vi "Analog IO Message - Continuous Pin Report.vi"(8 "error in (no error)":errorcluster, 9 "Enable Continuous Reporting?":bool, 10 "Pin Index":u8 format="%x", 11 "Refnum In":refnum<vi>) -> (0 "error out":errorcluster, 1 "Pin Value":u16, 2 "Pin Index Out":u8, 3 "Refnum Out":refnum<vi>)   [LabVIEW 2020, in "FirmataClient.lvlib"]
doc: "Allows requesting the state of a analog pin."
uses:
  FirmataClient.lvlib
  Controls/FirmataPinModes.ctl
panel:
  out "Pin Voltage":dbl
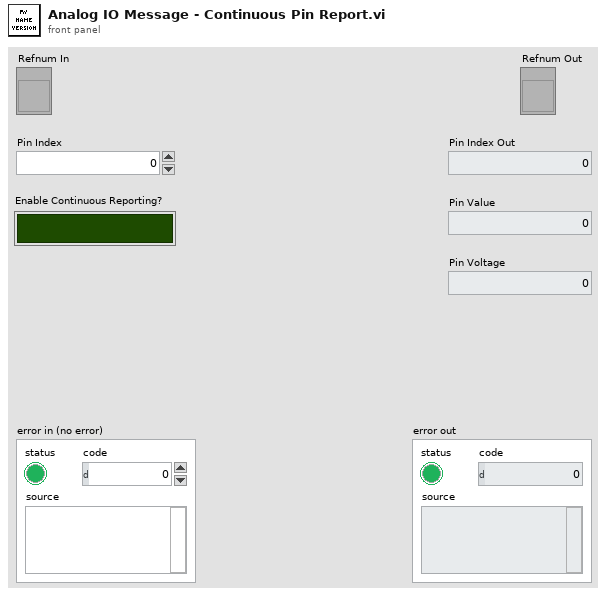
[diagram p1: front panel]
types:
  T1 = typedef "FirmataClient.lvlib/FirmataPinModes.ctl" = enum16{"DigitalInput", "DigitalOutput", "AnalogInput", "PWM", "Servo", "Shift", "I2C", "OneWire", "Stepper", "Encoder", "Serial", "InputPullup", "Extended.SPI", "Extended.Sonar", "Extended.Tone", "Extended.DHT"}
  T2 = typedef "FirmataClient.lvlib/FirmataProtocolConstants.ctl" = u16
  T3 = typedef "FirmataClient.lvlib/Parameters.ctl" = cluster{"Transport Parameters":T4, "Board Capabilities":map{i32, T6}}
  T4 = typedef "FirmataClient.lvlib/TransportParameters.ctl" = cluster{"Serial Communication":cluster{"Comport":refnum<visa-resource-name>, "No Response Timeout Ms":u32, "Response Complete Timeout Ms":u32, "Max Rx Length":u32, "Baud Rate":u32}, "Selected Transport":T5, "Initializer File Path":path, "Cleaner File Path":path, "Transporter File Path":path}
  T5 = typedef "FirmataClient.lvlib/SupportedTransports.ctl" = enum16{"Serial Communication Port"}
  T6 = typedef "FirmataClient.lvlib/FirmataPinCapabilitiesAndAnalogMapping.ctl" = cluster{"Supported Modes":T7[], "Analog Channel":u8, "Pin Name":string}
  T7 = typedef "FirmataClient.lvlib/FirmataPinCapability.ctl" = cluster{"PinMode":T1, "Resolution":u8}
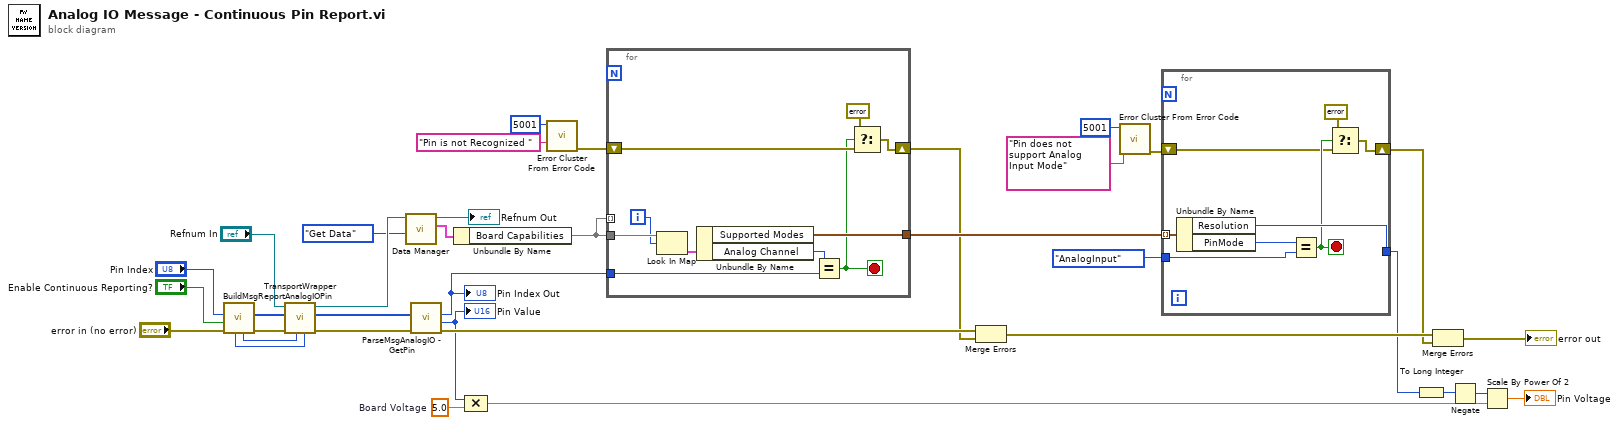
[diagram p0: block diagram]
diagram:
  w8 = 5.0  # Board Voltage
  n1 = call "BuildMsgReportAnalogIOPin.vi"("error in"="error in (no error)", "Enable Continuous Reporting?"="Enable Continuous Reporting?", "Pin Index"="Pin Index") -> ("error out"=w36:errorcluster, "AnalogIOMessage"=w31:u8[], "ReplyFirstByte"=w32:T2, "ReplyLength"=w33:i32)  [unwired: 5 in]
  n2 = call "TransportWrapper.vi"("ReplyLength"=w33, "ReplyFirstByte"=w32, "error in"=w36, "Message In"=w31, "Refnum In"="Refnum In") -> ("error out"=w28:errorcluster, "Message Out"=w27:u8[], "Refnum Out"=w26:refnum<vi>)  [unwired: 4 in]
  n3 = call "Data Manager.vi"("Mode"=enum16{"Store Data", "Get Data", "Cleanup"}."Get Data", "Refnum In"=w26) -> ("Data Out"=w23:T3, "Refnum Out"=→"Refnum Out":refnum<vi>)  [unwired: 7 in, 1 out]
  n4 = call "ParseMsgAnalogIO - GetPin.vi"("error in"=w28, "Message"=w27) -> ("error out"=w17:errorcluster, "Pin Value"=w9:u16, "Pin Index"=w4:u8)  [unwired: 7 in]
  "Pin Value" <- w9
  "Pin Index Out" <- w4
  n5 = Unbundle By Name(w23) -> ("Board Capabilities"=w5:map{i32, T6})
  n6 = Compound Arithmetic op=MULTIPLY(w9, w8) -> (w7:dbl)
  n7 = call <vilib>:"Error Cluster From Error Code.vi"("error message (\"\")"="Pin is not Recognized " ("error message (\"\")"), "error code (0)"=5001) -> ("error out"=w2:errorcluster)  [unwired: 7 in]
  n8 = for {
    tunnel: w5 -> [w46]
    tunnel: w5 -> [_] mode=indexing
    tunnel: w4 -> [w42]
    tunnel: [w41] -> w3
    shift-right: [w38] -> w1
    shift-left: w2 -> [w39]
    i -> [w45]
    stop <- w37 stop-if-true
    n9 = Look In Map(map=w46, key=w45) -> (value=w44:T6)  [unwired: 1 in, 1 out]
    n10 = Unbundle By Name(w44) -> ("Supported Modes"=w41:T7[], "Analog Channel"=w43:u8)
    n11 = Equal?(x=w43, y=w42) -> (x = y?=w37:bool)
    n12 = Select(t=errorcluster {"status"=FALSE, "code"=0, "source"=""}, s=w37, f=w39) -> (s? t:f=w38:errorcluster)
  }
  n13 = Merge Errors(w17, w1) -> (w15:errorcluster)
  n14 = call <vilib>:"Error Cluster From Error Code.vi"("error message (\"\")"="Pin does not support Analog Input Mode" ("error message (\"\")"), "error code (0)"=5001) -> ("error out"=w16:errorcluster)  [unwired: 7 in]
  n15 = for {
    tunnel: w3 -> [w54] mode=indexing
    tunnel: FirmataPinModes."AnalogInput" ("PinMode") -> [w52]
    tunnel: [w51] -> w11
    shift-right: [w48] -> w14
    shift-left: w16 -> [w49]
    stop <- w50 stop-if-true
    n16 = Unbundle By Name(w54) -> ("Resolution"=w51:u8, "PinMode"=w53:T1)
    n17 = Equal?(x=w53, y=w52) -> (x = y?=w50:bool)
    n18 = Select(t=errorcluster {"status"=FALSE, "code"=0, "source"=""}, s=w50, f=w49) -> (s? t:f=w48:errorcluster)
  }
  n19 = To Long Integer(number=w11) -> (32bit integer=w10:i32)
  n20 = Merge Errors(w15, w14) -> (→"error out":errorcluster)
  n21 = Negate(x=w10) -> (-x=w12:i32)
  n22 = Scale By Power Of 2(n=w12, x=w7) -> (x*2^n=→"Pin Voltage":dbl)
